vi "child 2 define test.vi"   [LabVIEW 2013, in "Unit Tests for Runner.lvclass"]
uses:
  Unit Tests for Runner.lvclass
  classes/Test/Test.lvclass
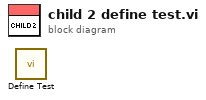
[diagram p0: block diagram]
diagram:
  n1 = call "Define Test.vi"() -> ()  [unwired: 11 in, 1 out]
